vi "Configure Timing.vi"(8 "error in (no error)":errorcluster, 11 "DAQmx Base CFG in":refnum<class "DAQmx Base CFG.lvclass">) -> (0 "error out":errorcluster, 3 "DAQmx Base CFG out":refnum<class "DAQmx Base CFG.lvclass">)   [LabVIEW 2023, in "DAQmx Base CFG.lvclass"]
uses:
  DAQmx Base CFG.lvclass
  Configuration/Configuration JSON/Configuration JSON Base/CFG JSON.lvclass
  3a10eacc-4dca-40d5-9fc9-a43ea3856a05.vi
  <vilib>/Utility/error.llb/Error Cluster From Error Code.vi
  <vilib>/ErrorRing/Error Ring.xnode
  <vilib>/DAQmx/configure/timing.llb/DAQmx Timing (Sample Clock).vi
  <vilib>/DAQmx/configure/timing.llb/DAQmx Timing (Implicit).vi
  D:/git/HAL/HAL GOOP4/Configuration JSON Base/CFG JSON.lvclass
  D:/git/HAL/HAL GOOP4/Interfaces/IConfigure/IConfigure.lvclass
  D:/git/HAL/HAL GOOP4/DAQmx/DAQmx Base CFG/DAQmx Base CFG.lvclass
panel:
  out "Active Edge":i32(ring)=10280 items=["Rising"=10280, "Falling"=10171]
  out "Sample Mode":i32(ring)=10178 items=["Finite Samples"=10178, "Continuous Samples"=10123, "Hardware Timed Single Point"=12522]
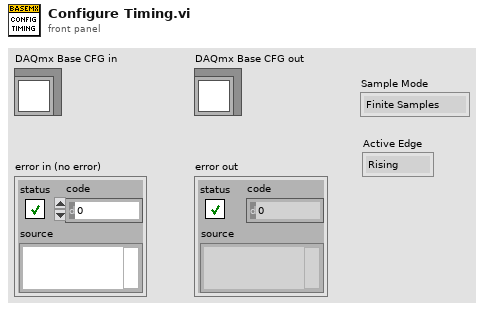
[diagram p1: front panel]
types:
  T1 = cluster{"Samples per Channel":i32, "Sample Mode":string, "Sample Rate":dbl, "Sample Clock Source":string, "Active Edge":string}
  T2 = typedef "LVStringsAndValuesArrayTypeDef_I32.ctl" = cluster{"String":string, "Value":i32}[]
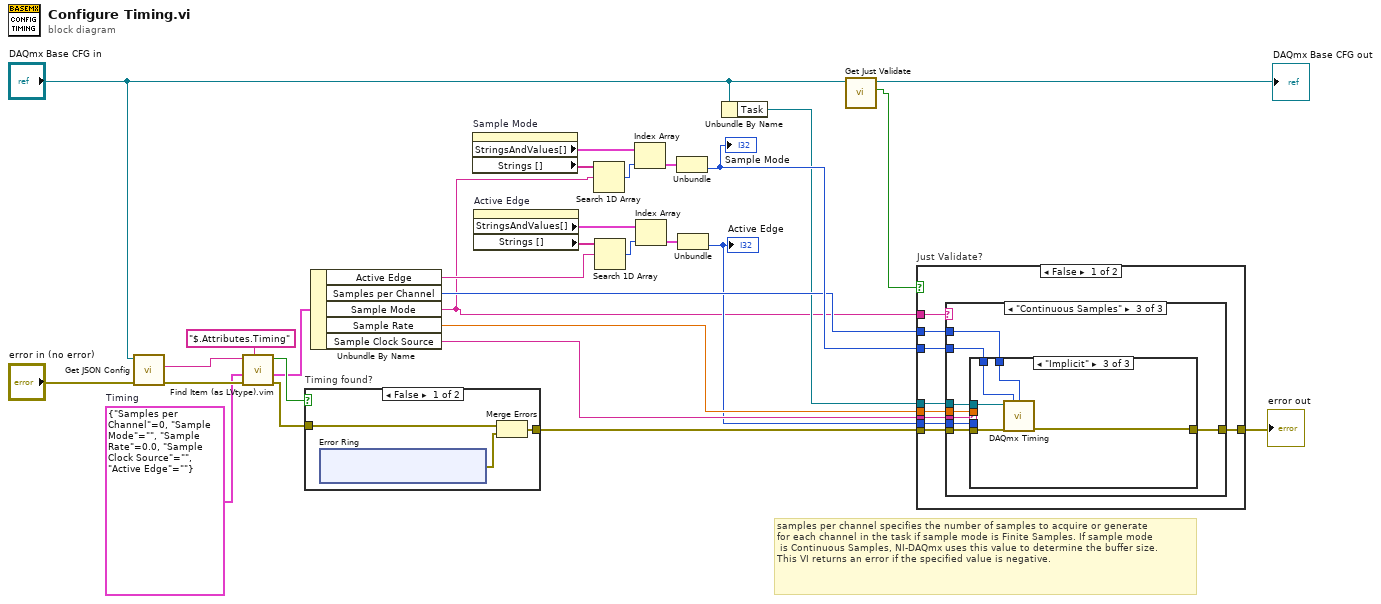
[diagram p0: block diagram]
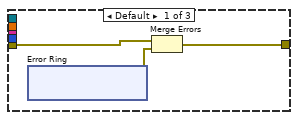
[diagram p2: hidden frame]
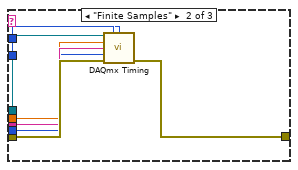
[diagram p3: hidden frame]
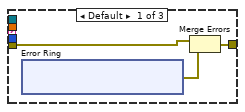
[diagram p4: hidden frame]
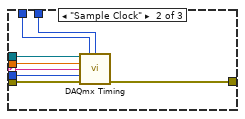
[diagram p5: hidden frame]
diagram:
  w26 = T1 {"Samples per Channel"=0, "Sample Mode"="", "Sample Rate"=0.0, "Sample Clock Source"="", "Active Edge"=""}  # Timing
  # "samples per channel specifies the number of samples to acquire or generate\nfor each channel in the task if sample mode is Finite Samples. If sample mode\n is Continuous Samples, NI-DAQmx uses this value to determine the buffer size.\nThis VI returns an error if the specified value is negative."
  n1 = call "Get JSON Config.vi"("error in (no error)"="error in (no error)", "CFG Base in"="DAQmx Base CFG in") -> ("error out"=w29:errorcluster, "<JSON>Config>"=w28:string)  [unwired: 7 in, 1 out]
  n2 = call "Find Item (as LVtype).vim"("$Path or Item Name"="$.Attributes.Timing", "error in (no error)"=w29, "Data Type and Default Value"=w26, "JSON"=w28) -> ("error out"=w24:errorcluster, "Data"=w19:T1, "Found"=w25:bool)  [unwired: 4 in, 1 out]
  n3 = case "Timing found?" shown="False" w25 {
    tunnel: w24 -> [w31 w38]
    tunnel: [w30 w38] -> w18
    frame False {
      n4 = xnode "Error Ring"() -> ("error out"=w32:errorcluster)
      n5 = Merge Errors(w31, w32) -> (w30:errorcluster)
    }
    frame True {
    }
  }
  n6 = Unbundle By Name(w19) -> ("Active Edge"=w7:string, "Samples per Channel"=w10:i32, "Sample Mode"=w6:string, "Sample Rate"=w12:dbl, "Sample Clock Source"=w17:string)
  n7 = property on="Sample Mode" class="Ring (strict)"() -> ("StringsAndValues[]"=w21:T2, "Strings []"=w20:string[])  [unwired: 2 in, 2 out]
  n8 = property on="Active Edge" class="Ring (strict)"() -> ("StringsAndValues[]"=w15:T2, "Strings []"=w16:string[])  [unwired: 2 in, 2 out]
  n9 = Search 1D Array(1D array=w20, element=w6) -> (index of element=w22:i32)  [unwired: 1 in]
  n10 = Search 1D Array(1D array=w16, element=w7) -> (index of element=w14:i32)  [unwired: 1 in]
  n11 = Index Array(array=w21, index=w22) -> (element=w23:cluster{"String":string, "Value":i32})
  n12 = Index Array(array=w15, index=w14) -> (element=w13:cluster{"String":string, "Value":i32})
  n13 = Unbundle(w23) -> ("Value"=w11:i32)  [unwired: 1 out]
  "Sample Mode" <- w11
  n14 = Unbundle(w13) -> ("Value"=w8:i32)  [unwired: 1 out]
  "Active Edge" <- w8
  n15 = Unbundle By Name("DAQmx Base CFG in") -> ("Task"=w9:refnum<k21>)
  n16 = call "Get Just Validate.vi"("CFG JSON Base in"="DAQmx Base CFG in") -> ("Just Validate"=w1:bool, "CFG JSON Base out"=→"DAQmx Base CFG out":refnum<class "DAQmx Base CFG.lvclass">)  [unwired: 8 in, 1 out]
  n17 = case "Just Validate?" shown="False" w1 {
    tunnel: w18 -> [w47 w93]
    tunnel: w17 -> [w46 _]
    tunnel: w12 -> [w45 _]
    tunnel: w11 -> [w44 _]
    tunnel: w10 -> [w43 _]
    tunnel: w9 -> [w42 _]
    tunnel: w8 -> [w41 _]
    tunnel: w6 -> [w40 _]
    tunnel: [w39 w93] -> w5
    frame False {
      n18 = case shown="\"Continuous Samples\"" w40 {
        tunnel: w47 -> [w49 w63 w71]
        tunnel: w46 -> [_ w62 w65]
        tunnel: w45 -> [_ w61 w70]
        tunnel: w44 -> [_ w60 w69]
        tunnel: w43 -> [_ w59 w64]
        tunnel: w42 -> [_ w58 w68]
        tunnel: [w50 w57 w67] -> w39
        tunnel: w41 -> [_ w56 w66]
        frame Default {
          n19 = xnode "Error Ring"() -> ("error out"=w48:errorcluster)
          n20 = Merge Errors(w49, w48) -> (w50:errorcluster)
        }
        frame "Finite Samples" {
          n21 = call-poly <vilib>:"DAQmx Timing.vi"("task/channels in"=w58, "sample mode"=w60, "samples per channel"=w59, "rate"=w61, "source"=w62, "active edge"=w56, "error in"=w63) -> ("error out"=w57:errorcluster)  [unwired: 7 in, 1 out]
        }
        frame "Continuous Samples" {
          n22 = case shown="\"Implicit\"" w65 {
            selector: w65 -> [_ w81 _]
            tunnel: w71 -> [w73 w87 w92]
            tunnel: w70 -> [_ w86 _]
            tunnel: w69 -> [_ w85 w89]
            tunnel: w68 -> [_ w84 w90]
            tunnel: [w74 w83 w91] -> w67
            tunnel: w66 -> [_ w82 _]
            tunnel: w64 -> [_ w80 w88]
            frame Default {
              n23 = xnode "Error Ring"() -> ("error out"=w72:errorcluster)
              n24 = Merge Errors(w73, w72) -> (w74:errorcluster)
            }
            frame "Sample Clock" {
              n25 = call-poly <vilib>:"DAQmx Timing.vi"("task/channels in"=w84, "sample mode"=w85, "samples per channel"=w80, "rate"=w86, "source"=w81, "active edge"=w82, "error in"=w87) -> ("error out"=w83:errorcluster)  [unwired: 7 in, 1 out]
            }
            frame "Implicit" {
              n26 = call-poly <vilib>:"DAQmx Timing.vi"("task/channels in"=w90, "sample mode"=w89, "samples per channel"=w88, "error in"=w92) -> ("error out"=w91:errorcluster)  [unwired: 10 in, 1 out]
            }
          }
        }
      }
    }
    frame True {
    }
  }
  "error out" <- w5
